vi "GraphsDirectory.vi"() -> (3 "dup path":path)   [LabVIEW 2013]
uses:
  Global.vi
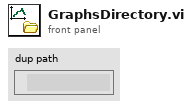
[diagram p1: front panel]
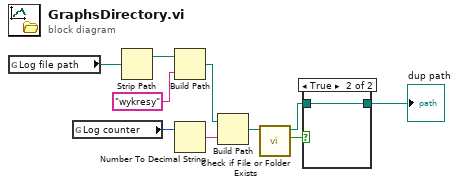
[diagram p0: block diagram]
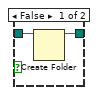
[diagram p2: hidden frame]
diagram:
  n1 = global read "Global.vi" "Log file path"() -> (w3:path)
  n2 = global read "Global.vi" "Log counter"() -> (w5:i32)
  n3 = Strip Path(path=w3) -> (stripped path=w2:path)  [unwired: 1 out]
  n4 = Build Path(base path=w2, name or relative path="wykresy") -> (appended path=w4:path)
  n5 = Number To Decimal String(number=w5) -> (decimal integer string=w6:string)  [unwired: 1 in]
  n6 = Build Path(base path=w4, name or relative path=w6) -> (appended path=w7:path)
  n7 = call <vilib>:"Check if File or Folder Exists.vi"("path"=w7) -> ("file or folder exists?"=w8:bool, "dup path"=w9:path)  [unwired: 8 in, 1 out]
  n8 = case shown="True" w8 {
    tunnel: w9 -> [w12 w13]
    tunnel: [w11 w13] -> w10
    frame False {
      n9 = Create Folder(path (use dialog)=w12) -> (created path=w11:path)  [unwired: 2 in, 2 out]
    }
    frame True {
    }
  }
  "dup path" <- w10
